vi "Save_File_Sample_Setup.vi"(8 "Error In":errorcluster, 9 "input cluster":T1={"system"={"info"={"menuSelect"=100, "version"=1000, "serial"="Test Sample", "captureActive"=FALSE, "captureBegin"=FALSE, "emptyAndRefill"=FALSE}, "userInfo"={"operatorName"="MRJ", "date"=timestamp(2713993200 s since 1904-01-01)}, "camera"={"exposureTime"=1, "aperture"=enum."Item 0", "framerate"=1, "framerateMax"=500, "legacyAttributes"=FALSE}}, "connections"={"arduino"={"connection"="MRJ", "status"=FALSE, "openState"=FALSE, "emptyStart"=500}, "pump"={"connection"="MRJ", "status"=FALSE, "command"="", "dispenseSpeed"=500, "flushSize"=100}, "camera"={"cam1"={"connection"="", "status"=FALSE}, "cam2"={"connection"="", "status"=FALSE}}}, "queue"={"process"={"cam1"=refnum, "cam2"=refnum, "queueSize"=0}, "save"={"cam1"=refnum, "cam2"=refnum, "queueSize"=0}, "overloadThreshold"=0}, "imageProcess"={"cam1"={"preAllocation"={"image"=refnum, "originalDisplay"=refnum, "originalRgb"=refnum, "binary"=refnum, "save"=refnum, "calibrationFull"=refnum, "calibrationDetect"=refnum}, "calibration"={"pathFull"=path "C:/Users/au540322/Desktop/IHS_Project/images/Debris/Debris_0/Debris_0_2019_06_01-23-32-49-686.PNG", "pathDetect"=path "C:/Users/au540322/Desktop/IHS_Project/images/Debris/Debris_0/Debris_0_2019_06_01-23-32-49-686.PNG", "ROI"={"Left"=0, "Top"=0, "Right"=0, "Bottom"=0, "Rotation"=0.0}}}, "cam2"={"preAllocation"={"image"=refnum, "originalDisplay"=refnum, "originalRgb"=refnum, "binary"=refnum, "save"=refnum, "calibrationFull"=refnum, "calibrationDetect"=refnum}, "calibration"={"pathFull"=path "C:/Users/au540322/Desktop/IHS_Project/images/Debris/Debris_0/Debris_0_2019_06_01-23-32-49-686.PNG", "pathDetect"=path "C:/Users/au540322/Desktop/IHS_Project/images/Debris/Debris_0/Debris_0_2019_06_01-23-32-49-686.PNG", "ROI"={"Left"=0, "Top"=0, "Right"=0, "Bottom"=0, "Rotation"=0.0}}}, "process"={"planeExtract"=refnum, "planeSubtract"=refnum, "cropMask"=refnum}, "detection"={"sampleTimeout"=200, "sizeThreshold"=500, "detectionRegionPct"=0.0}}, "sampleData"={"sampleId"="", "projectId"="", "voucherID"="", "speciesName"="", "collectionDate"=timestamp(2713993200 s since 1904-01-01), "sampleStation"="", "location"="", "lat"=0.0, "lon"=0.0, "determiner"="", "sex"="", "otherNotes"=""}, "Session In"=""} {"sampleData"."collectionDate" format="%<%Y-%m-%d>T"; "imageProcess"."detection"."sizeThreshold" min=1; "imageProcess"."cam2"."calibration"."ROI"."Rotation" format="%.2f"; "imageProcess"."cam2"."calibration"."ROI"."Left" scale=0.0..1024.0; "imageProcess"."cam2"."calibration"."ROI"."Right" scale=0.0..1024.0; "imageProcess"."cam1"."calibration"."ROI"."Rotation" format="%.2f"; "imageProcess"."cam1"."calibration"."ROI"."Left" scale=0.0..1024.0; "imageProcess"."cam1"."calibration"."ROI"."Right" scale=0.0..1024.0; "queue"."overloadThreshold" min=1; "queue"."save"."queueSize" min=1; "queue"."process"."queueSize" min=1; "connections"."pump"."flushSize" min=1; "connections"."pump"."dispenseSpeed" min=1; "system"."camera"."framerateMax" min=1; "system"."userInfo"."date" format="%<%Y-%m-%dT%H:%M:%S+%z>T"; "system"."info"."version" items=["Standard", "XL"]; "system"."info"."menuSelect" items=["Session Data", "Extended Setup", "Buffer", "Camera", "Dispenser", "Stats", "Connections"]}, 11 "Sample Subfolder Name":string) -> (0 "Error Out":errorcluster)   [LabVIEW 2022 SP3]
doc: "Save a file containing current sample setup information:\n\nCamera settings\n- Exposure Time [µs]\n- Light Intensity [%]\n- Sample Frequency [FPS]\n\nOperator\n- Name\n- Sample Notes/Description\n\nDate\n- DDMMYYYY"
uses:
  <vilib>/Utility/config.llb/NI_LVConfig.lvlib
  <vilib>/Utility/config.llb/Write Key (String).vi
  <vilib>/userdefined/High Color/IMAQdx.ctl
  <vilib>/vision/Image Controls.llb/IMAQ Image.ctl
  controls/Data.ctl
panel:
  out "?":errorcluster
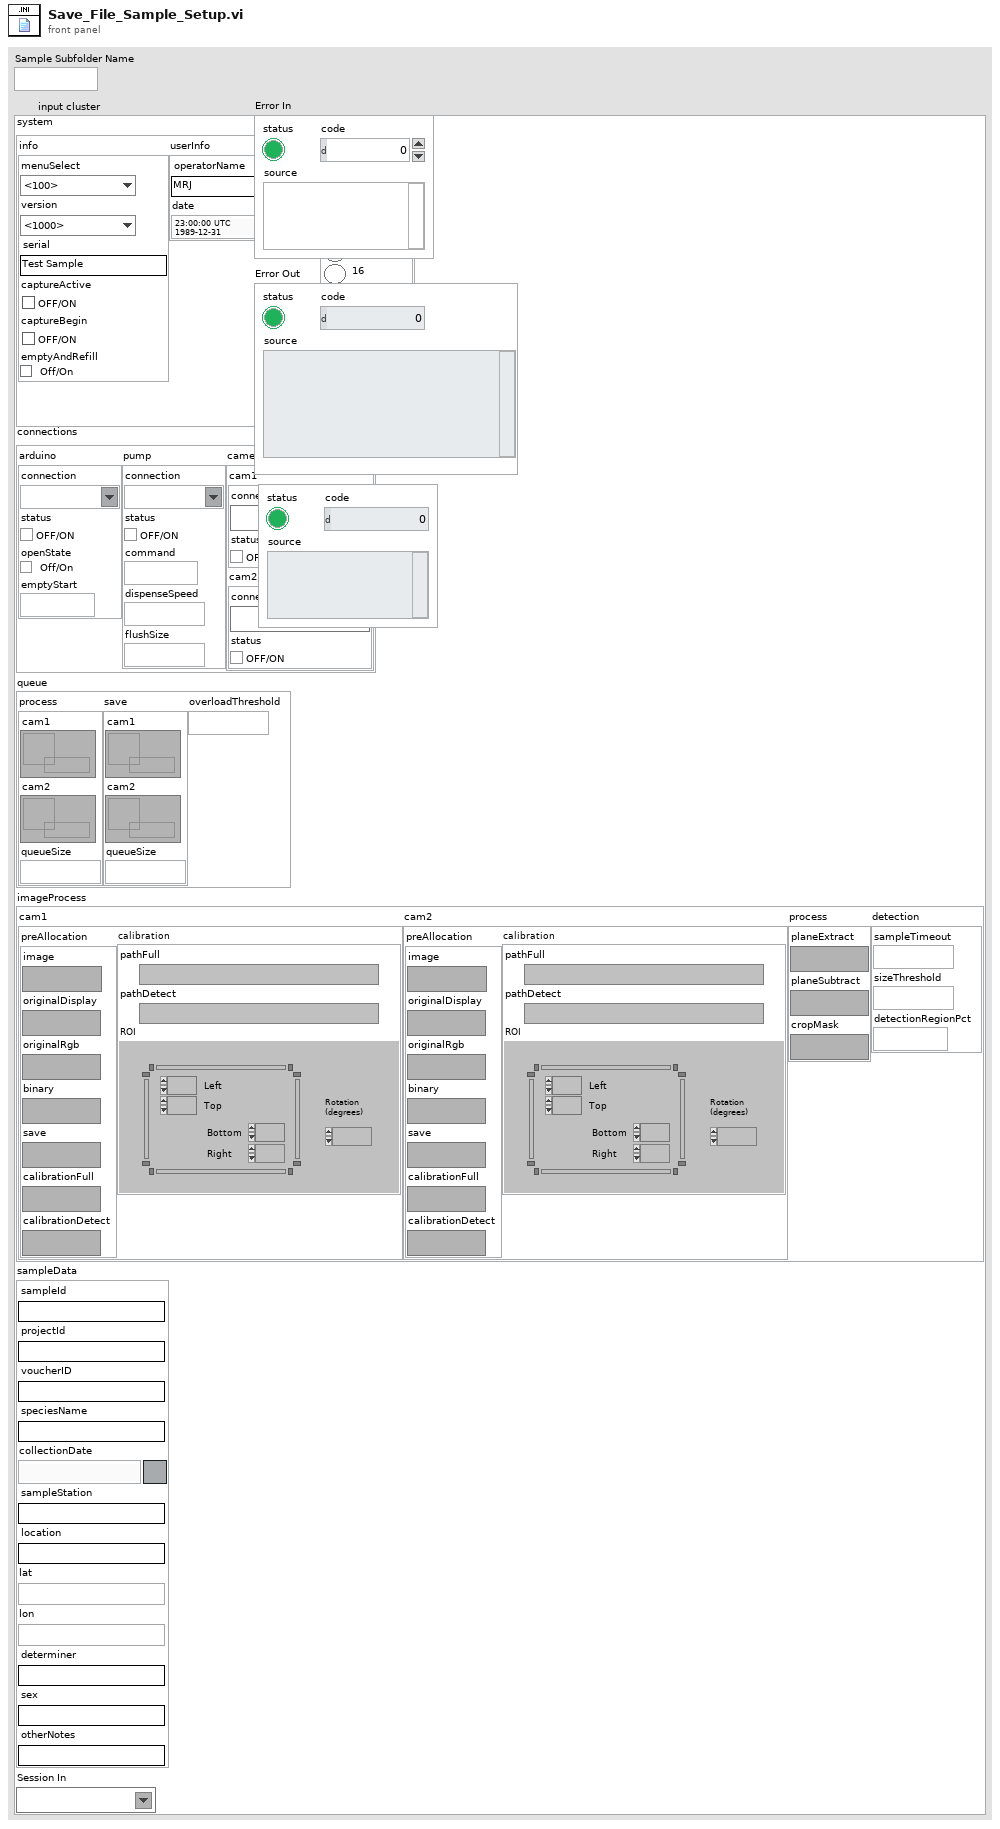
[diagram p1: front panel]
types:
  T1 = typedef "Data.ctl" = cluster{"system":cluster{"info":cluster{"menuSelect":u16, "version":u16, "serial":string, "captureActive":bool, "captureBegin":bool, "emptyAndRefill":bool}, "userInfo":cluster{"operatorName":string, "date":timestamp}, "camera":cluster{"exposureTime":i32, "aperture":enum32{"Item 0", "Item 1", "Item 2", "Item 3"}, "framerate":i32, "framerateMax":i32, "legacyAttributes":bool}}, "connections":cluster{"arduino":cluster{"connection":refnum<visa-resource-name>, "status":bool, "openState":bool, "emptyStart":u32}, "pump":cluster{"connection":refnum<visa-resource-name>, "status":bool, "command":string, "dispenseSpeed":i32, "flushSize":i32}, "camera":cluster{"cam1":cluster{"connection":T2, "status":bool}, "cam2":cluster{"connection":T2, "status":bool}}}, "queue":cluster{"process":cluster{"cam1":refnum<queue>, "cam2":refnum<queue>, "queueSize":i32}, "save":cluster{"cam1":refnum<queue>, "cam2":refnum<queue>, "queueSize":i32}, "overloadThreshold":i32}, "imageProcess":cluster{"cam1":cluster{"preAllocation":cluster{"image":T3, "originalDisplay":T3, "originalRgb":T3, "binary":T3, "save":T3, "calibrationFull":T3, "calibrationDetect":T3}, "calibration":cluster{"pathFull":path, "pathDetect":path, "ROI":T4}}, "cam2":cluster{"preAllocation":cluster{"image":T3, "originalDisplay":T3, "originalRgb":T3, "binary":T3, "save":T3, "calibrationFull":T3, "calibrationDetect":T3}, "calibration":cluster{"pathFull":path, "pathDetect":path, "ROI":T4}}, "process":cluster{"planeExtract":T3, "planeSubtract":T3, "cropMask":T3}, "detection":cluster{"sampleTimeout":i32, "sizeThreshold":i32, "detectionRegionPct":dbl}}, "sampleData":cluster{"sampleId":string, "projectId":string, "voucherID":string, "speciesName":string, "collectionDate":timestamp, "sampleStation":string, "location":string, "lat":dbl, "lon":dbl, "determiner":string, "sex":string, "otherNotes":string}, "Session In":T2}
  T2 = typedef "IMAQdx.ctl" = refnum<k21>
  T3 = typedef "IMAQ Image.ctl" = refnum<image>
  T4 = typedef "IMAQ Rectangle" = cluster{"Left":i32, "Top":i32, "Right":i32, "Bottom":i32, "Rotation":dbl}
  T5 = typedef "NI_LVConfig.lvlib/Config Data RefNum.ctl" = refnum<k1>
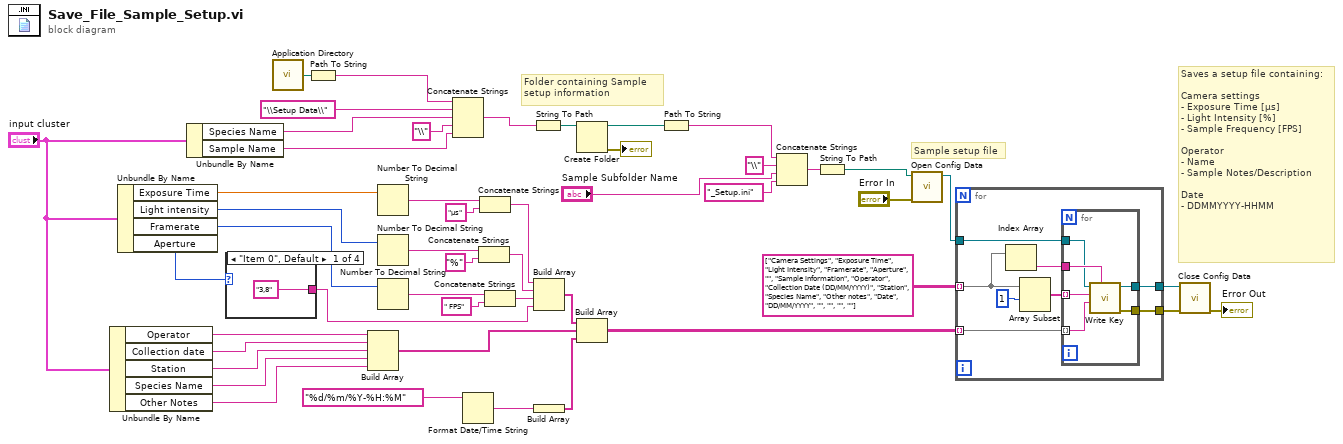
[diagram p0: block diagram]
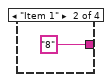
[diagram p2: hidden frame]
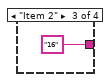
[diagram p3: hidden frame]
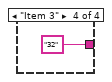
[diagram p4: hidden frame]
diagram:
  # "Saves a setup file containing:\n\nCamera settings\n- Exposure Time [µs]\n- Light Intensity [%]\n- Sample Frequency [FPS]\n\nOperator\n- Name\n- Sample Notes/Description\n\nDate\n- DDMMYYYY-HHMM"
  # "Sample setup file"
  # "Folder containing Sample \nsetup information"
  n1 = Unbundle By Name("input cluster") -> ("Operator"=w8:string, "Collection date"=w7:string, "Station"=w6:string, "Species Name"=w5:string, "Other Notes"=w4:string)
  n2 = Unbundle By Name("input cluster") -> ("Exposure Time"=w27:dbl, "Light intensity"=w26:i32, "Framerate"=w15:i32, "Aperture"=w3:enum32{"Item 0", "Item 1", "Item 2", "Item 3"})
  n3 = Unbundle By Name("input cluster") -> ("Species Name"=w13:string, "Sample Name"=w11:string)
  n4 = case shown="\"Item 0\", Default" w3 {
    tunnel: ["3,8" "8" "16" "32"] -> w2
    frame "Item 0", Default {
    }
    frame "Item 1" {
    }
    frame "Item 2" {
    }
    frame "Item 3" {
    }
  }
  n5 = call <vilib>:"Application Directory.vi"() -> ("Application Directory"=w37:path)
  n6 = Path To String(path=w37) -> (string=w35:string)
  n7 = Build Array(w8, w7, w6, w5, w4) -> (w14:string[])
  n8 = Number To Decimal String(number=w27) -> (decimal integer string=w21:string)  [unwired: 1 in]
  n9 = Number To Decimal String(number=w26) -> (decimal integer string=w23:string)  [unwired: 1 in]
  n10 = Number To Decimal String(number=w15) -> (decimal integer string=w18:string)  [unwired: 1 in]
  n11 = Concatenate Strings(w35, "\\Setup Data\\" ("string"), w13, "\\" ("string"), w11) -> (w10:string)
  n12 = Format Date/Time String(time format string (%c)="%d/%m/%Y-%H:%M") -> (date/time string=w38:string)  [unwired: 2 in]
  n13 = Concatenate Strings(w23, "%" ("string")) -> (w22:string)
  n14 = Concatenate Strings(w21, "µs" ("string")) -> (w19:string)
  n15 = Concatenate Strings(w18, " FPS" ("string")) -> (w17:string)
  n16 = String To Path(string=w10) -> (path=w34:path)
  n17 = Build Array(w19, w22, w17, w2) -> (w48:string[])
  n18 = Build Array(w38) -> (w39:string[])
  n19 = Create Folder(path (use dialog)=w34) -> (created path=w32:path, error out=→"?":errorcluster)  [unwired: 2 in, 1 out]
  n20 = Build Array(w48, w14, w39) -> (w47:string[][])
  n21 = Path To String(path=w32) -> (string=w31:string)
  n22 = Concatenate Strings(w31, "\\" ("string"), "Sample Subfolder Name", "_Setup.ini" ("string")) -> (w41:string)
  n23 = String To Path(string=w41) -> (path=w43:path)
  n24 = call <vilib>:"Open Config Data.vi"("error in (no error)"="Error In", "configuration file path"=w43) -> ("refnum"=w44:T5)  [unwired: 7 in, 2 out]
  n25 = for {
    tunnel: string[][] [["Camera Settings", "Exposure Time", "Light Intensity", "Framerate", "Aperture", ""], ["Sample information", "Operator", "Collection Date (DD/MM/YYYY)", "Station", "Species Name", "Other notes"], ["Date", "DD/MM/YYYY", "", "", "", ""]] ("appended array") -> [w59] mode=indexing
    tunnel: w47 -> [w57] mode=indexing
    tunnel: [w55] -> w46
    tunnel: [w54] -> w45
    tunnel: w44 -> [w53]
    n26 = Index Array(array=w59) -> (element=w58:string)  [unwired: 1 in]
    n27 = Array Subset(array=w59, index=1) -> (w56:string[])  [unwired: 1 in]
    n28 = for {
      tunnel: w58 -> [w66]
      tunnel: w57 -> [w65] mode=indexing
      tunnel: w56 -> [w64] mode=indexing
      tunnel: [w63] -> w55
      tunnel: [w62] -> w54
      tunnel: w53 -> [w61]
      n29 = call-poly <vilib>:"Write Key.vi"("section"=w66, "value"=w65, "key"=w64, "refnum"=w61) -> ("error out"=w62:errorcluster, "refnum out"=w63:T5)  [unwired: 5 in, 1 out]
    }
  }
  n30 = call <vilib>:"Close Config Data.vi"("error in (no error)"=w45, "refnum"=w46) -> ("error out"=→"Error Out":errorcluster)  [unwired: 8 in, 1 out]
